vi "Set speed graph behaviour ctrl.vi"(8 "error in":errorcluster, 11 "Exporter's ctrl refs":T1) -> (0 "error out":errorcluster)   [LabVIEW 2020]
uses:
  Typedefs/8-bit video export window ctrl refs.ctl
  Patch-Vol video generator/Typedefs/Bright-Contr-Gamma cluster.ctl
  Typedefs/Speed graph behaviour enum.ctl
  Functional Imaging Viewer/Typedefs/Get-Set-Clear Control.ctl
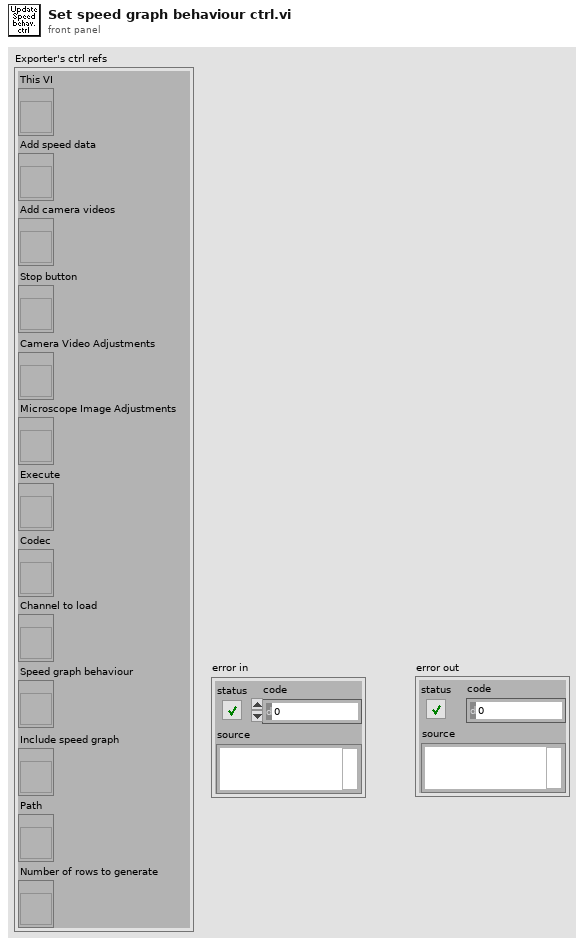
[diagram p1: front panel]
types:
  T1 = typedef "8-bit video export window ctrl refs.ctl" = cluster{"This VI":refnum<vi>, "Add speed data":refnum<vi>, "Add camera videos":refnum<vi>, "Stop button":refnum<vi>, "Camera Video Adjustments":refnum<vi>, "Microscope Image Adjustments":refnum<vi>, "Execute":refnum<vi>, "Codec":refnum<vi>, "Channel to load":refnum<vi>, "Speed graph behaviour":refnum<vi>, "Include speed graph":refnum<vi>, "Number of rows to generate":refnum<vi>, "Path":refnum<vi>}
  T2 = typedef "Get-Set-Clear Control.ctl" = enum16{"Get", "Set", "Clear"}
  T3 = typedef "Speed graph behaviour enum.ctl" = enum16{"Scrolling data", "Scrolling cursor"}
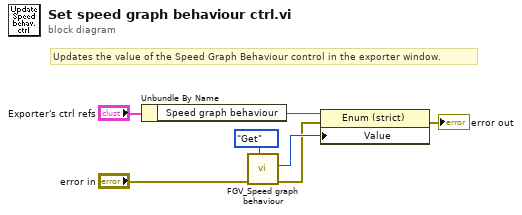
[diagram p0: block diagram]
diagram:
  # "Updates the value of the Speed Graph Behaviour control in the exporter window."
  n1 = Unbundle By Name("Exporter's ctrl refs") -> ("Speed graph behaviour"=w5:refnum<vi>)
  n2 = call "FGV_Speed graph behaviour.vi"("Function"=Get-Set-Clear_Control."Get", "error in (no error)"="error in") -> ("error out"=w2:errorcluster, "Speed graph behaviour"=w4:T3)  [unwired: 8 in]
  n3 = property on="Property Node" class="Enum (strict)"(reference=w5, error in=w2, "Value"=w4) -> (error out=→"error out":errorcluster)  [unwired: 1 out]
